vi "Test-SparkMax.vi"() -> ()   [LabVIEW 2023]
doc: "This VI implements the framework and scheduler for your robotics program. It should not be necessary to modify the framework. You are expected to add your code to the VIs called from Robot Main - the ones located in the Team Code folder within the project."
uses:
  Robot Global Data.vi
  <vilib>/Rock Robotics/WPI/DriverStation/WPI_DriverStationRobotMode2.ctl
  <vilib>/Rock Robotics/WPI/ThirdParty/REV Robotics/REVLib/Typedef/Spark MAX Limit Direction.ctl
  <vilib>/Rock Robotics/WPI/ThirdParty/REV Robotics/REVLib/Typedef/Spark MAX Limit Switch Polarity.ctl
panel:
  out "Loop Count":i32
  in  "Invert":bool
  in  "CAN Device Number":u8=1
  in  "Out-ut +/- 1.0":dbl
  out "Sensor Velocity  (REV/MIN)":dbl
  out "Sensor Position (REV)":dbl
  out "Hard Limit Rev":bool
  out "Hard Limit Fwd":bool
  in  "Rev Enabled":bool=TRUE
  in  "Rev Polarity":T1
  in  "Fwd Enabled":bool=TRUE
  in  "Fwd Polarity":T1
  in  "Finish":bool
  # "Set before starting\nProgram"
  # "Spark Max Test Program"
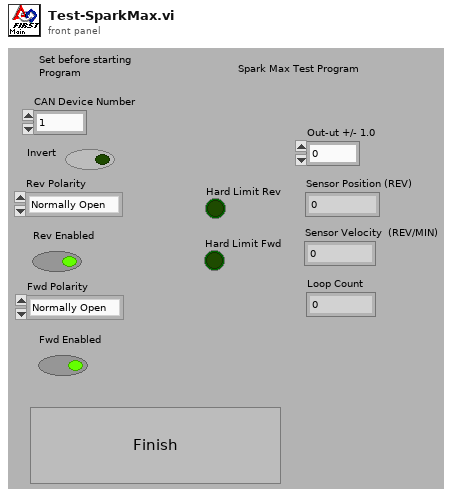
[diagram p1: front panel]
types:
  T1 = typedef "Spark MAX Limit Switch Polarity.ctl" = enum16{"Normally Open", "Normally Closed"}
  T2 = typedef "Spark MAX Limit Direction.ctl" = enum16{"Forward Limit", "Reverse Limit"}
  T3 = typedef "WPI_DriverStationRobotMode2.ctl" = enum16{"Autonomous Disabled", "Autonomous Enabled", "Teleop Disabled", "Teleop Enabled", "Disconnected", "Finish", "Test Disabled", "Test Enabled", "Emergency Stopped"}
  T4 = typedef "WPI_MotorControlDeviceRef.ctl" = cluster{"DeviceStatus":errorcluster, "Type":T5, "PWM":cluster{"PWM Channel":T6, "DeadBand":T7}, "CAN":cluster{"Device Number":u8, "SetOutput VI Ref":variant, "GetOutput VI Ref":variant, "Enable VI Ref":variant, "Disable VI Ref":variant, "Data":variant}, "Invert":bool, "DIO PWM":cluster{"PWM \"Enable\" Channel":T6, "DIOChannel":T8, "PWM Rate":dbl}}
  T5 = typedef "WPI_MotorControlType.ctl" = enum16{"PWM", "CAN", "DIO PWM"}
  T6 = typedef "FPGA_DIOPWMChannel.ctl" = enum8{"PWM 0", "PWM 1", "PWM 2", "PWM 3", "PWM 4", "PWM 5", "PWM 6", "PWM 7", "PWM 8", "PWM 9", "PWM MXP 0", "PWM MXP 1", "PWM MXP 2", "PWM MXP 3", "PWM MXP 4", "PWM MXP 5", "PWM MXP 6", "PWM MXP 7", "PWM MXP 8", "PWM MXP 9", "Invalid"}
  T7 = typedef "WPI_PWMDeadband.ctl" = cluster{"Name":string, "maxPositivePwm":i32, "minPositivePwm":i32, "centerPwm":i32, "maxNegativePwm":i32, "minNegativePwm":i32, "angularRange":u16}
  T8 = typedef "FPGA_DIOChannel.ctl" = enum8{"DIO 0", "DIO 1", "DIO 2", "DIO 3", "DIO 4", "DIO 5", "DIO 6", "DIO 7", "DIO 8", "DIO 9", "DIO MXP 0", "DIO MXP 1", "DIO MXP 2", "DIO MXP 3", "DIO MXP 4", "DIO MXP 5", "DIO MXP 6", "DIO MXP 7", "DIO MXP 8", "DIO MXP 9", "DIO MXP 10", "DIO MXP 11", "DIO MXP 12", "DIO MXP 13", "DIO MXP 14", "DIO MXP 15", "SPI Port CS1", "SPI Port CS2", "SPI Port CS3", "SPI Port MISO", "SPI Port MOSI", "Invalid"}
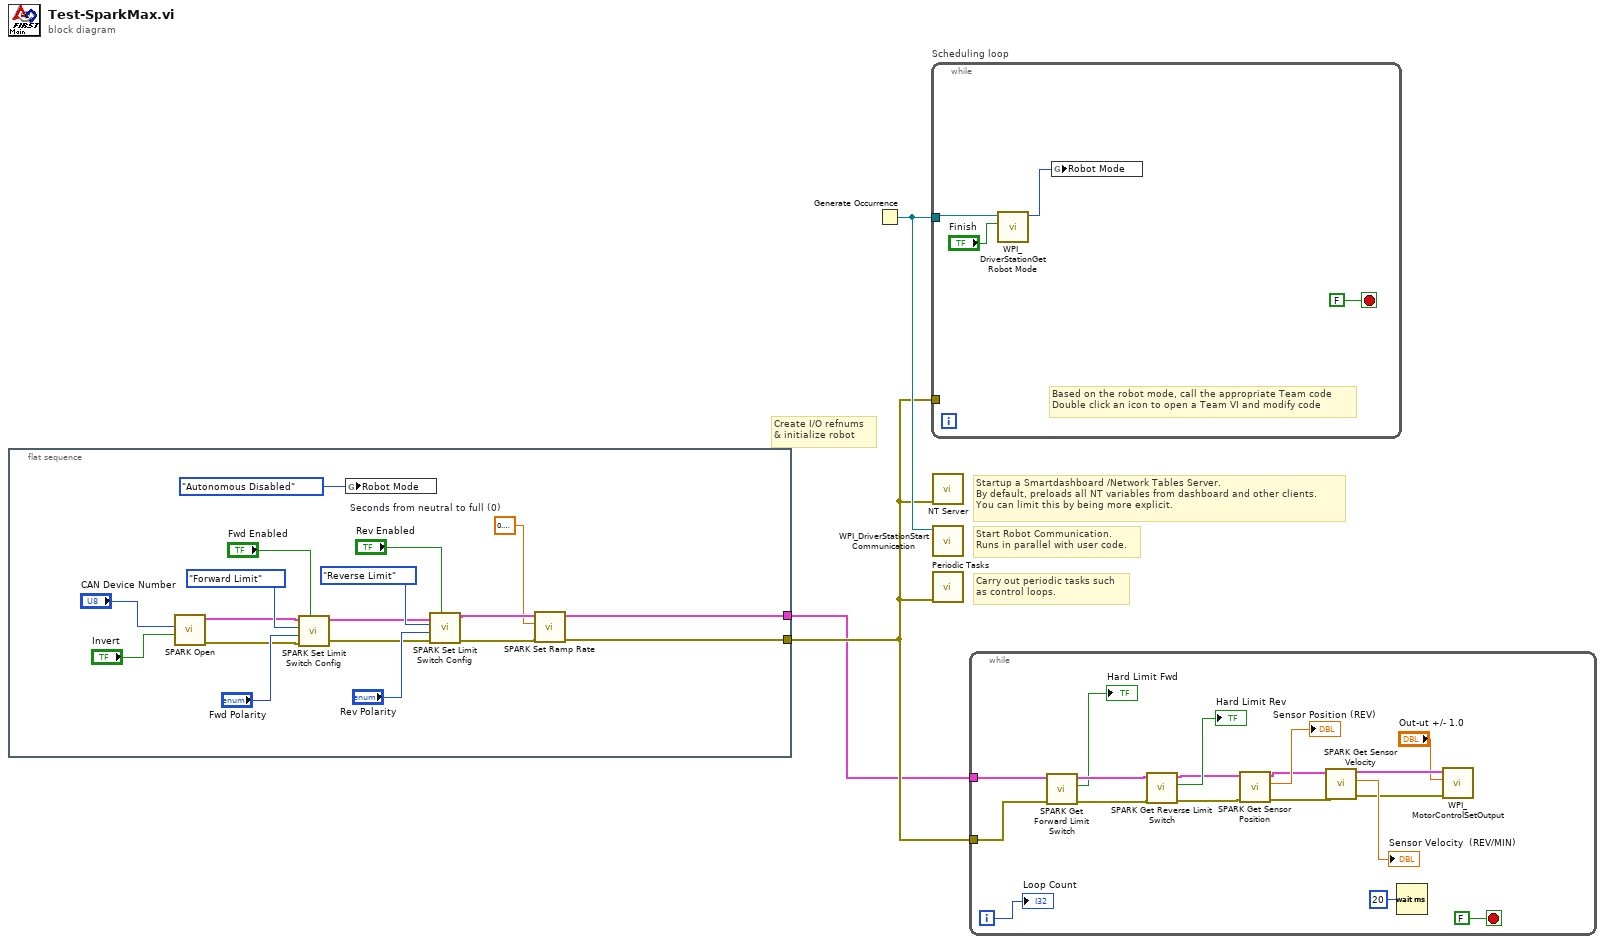
[diagram p0: block diagram]
diagram:
  # "Startup a Smartdashboard /Network Tables Server.\nBy default, preloads all NT variables from dashboard and other clients.\nYou can limit this by being more explicit."
  # "Carry out periodic tasks such\nas control loops."
  # "Create I/O refnums\n& initialize robot"
  # "Start Robot Communication.\nRuns in parallel with user code."
  n1 = flat-sequence {
    tunnel: [w7] -> w2
    tunnel: [w6] -> w1
    frame #0 {
      w9 = sgl 0.1  # Seconds from neutral to full (0)
      n2 = call <vilib>:"SPARK Open.vi"("Invert"="Invert", "Device Number"="CAN Device Number") -> ("error out"=w13:errorcluster, "MotorControlDeviceRef"=w14:T4)  [unwired: 8 in]
      n3 = call <vilib>:"SPARK Set Limit Switch Config.vi"("Enabled? (T)"="Fwd Enabled", "error in (no error)"=w13, "Polarity (Normally Open)"="Fwd Polarity", "Limit Switch"=Spark_MAX_Limit_Direction."Forward Limit", "MotorControlDeviceRef in"=w14) -> ("error out"=w11:errorcluster, "MotorControlDeviceRef out"=w12:T4)  [unwired: 5 in]
      n4 = global write "Robot Global Data.vi" "Robot Mode"(WPI_DriverStationRobotMode2."Autonomous Disabled" ("Robot Mode")) -> ()
      n5 = call <vilib>:"SPARK Set Limit Switch Config.vi"("Enabled? (T)"="Rev Enabled", "error in (no error)"=w11, "Polarity (Normally Open)"="Rev Polarity", "Limit Switch"=Spark_MAX_Limit_Direction."Reverse Limit", "MotorControlDeviceRef in"=w12) -> ("error out"=w8:errorcluster, "MotorControlDeviceRef out"=w10:T4)  [unwired: 5 in]
      n6 = call <vilib>:"SPARK Set Ramp Rate.vi"("error in (no error)"=w8, "Seconds from neutral to full (0)"=w9, "MotorControlDeviceRef in"=w10) -> ("error out"=w7:errorcluster, "MotorControlDeviceRef"=w6:T4)  [unwired: 7 in]
    }
  }
  n7 = Generate Occurrence() -> (w3:refnum<k4>)
  n8 = while "Scheduling loop" {
    tunnel: w3 -> [w25]
    tunnel: w2 -> [_]
    stop <- FALSE stop-if-true
    # "Based on the robot mode, call the appropriate Team code\nDouble click an icon to open a Team VI and modify code"
    n9 = call <vilib>:"WPI_DriverStationGet Robot Mode.vi"("Finish"="Finish", "DS Occurrence"=w25) -> ("Robot Mode"=w23:T3)  [unwired: 9 out]
    n10 = global write "Robot Global Data.vi" "Robot Mode"(w23) -> ()
  }
  n11 = call <vilib>:"NT Server.vi"("error in (no error)"=w2) -> ()  [unwired: 10 in, 1 out]
  n12 = call <vilib>:"WPI_DriverStationStart Communication.vi"("occurrence"=w3) -> ()  [unwired: 2 in, 9 out]
  n13 = call "Periodic Tasks.vi"("error in"=w2) -> ()  [unwired: 1 in, 10 out]
  n14 = while {
    tunnel: w2 -> [w40]
    tunnel: w1 -> [w41]
    i -> [w26]
    stop <- FALSE stop-if-true
    n15 = call <vilib>:"SPARK Get Forward Limit Switch.vi"("error in (no error)"=w40, "MotorControlDevRef in"=w41) -> ("error out"=w38:errorcluster, "Hard Limit Fwd"=→"Hard Limit Fwd":bool, "MotorControlDevRef out"=w39:T4)  [unwired: 6 in, 1 out]
    n16 = call <vilib>:"SPARK Get Reverse Limit Switch.vi"("error in (no error)"=w38, "MotorControlDevRef in"=w39) -> ("error out"=w35:errorcluster, "Hard Limit Rev"=→"Hard Limit Rev":bool, "MotorControlDevRef out"=w34:T4)  [unwired: 6 in, 1 out]
    n17 = call <vilib>:"SPARK Get Sensor Position.vi"("error in (no error)"=w35, "MotorControlDevRef in"=w34) -> ("error out"=w31:errorcluster, "Sensor Position"=→"Sensor Position (REV)":dbl, "MotorControlDevRef out"=w32:T4)  [unwired: 6 in, 1 out]
    n18 = call <vilib>:"SPARK Get Sensor Velocity.vi"("error in (no error)"=w31, "MotorControlDevRef in"=w32) -> ("error out"=w28:errorcluster, "Sensor Velocity"=→"Sensor Velocity  (REV/MIN)":dbl, "MotorControlDevRef out"=w30:T4)  [unwired: 6 in, 1 out]
    n19 = Wait (ms)(milliseconds to wait=u32 20) -> ()  [unwired: 1 out]
    n20 = call <vilib>:"WPI_MotorControlSetOutput.vi"("error in (no error)"=w28, "Output"="Out-ut +/- 1.0", "MotorControlDevRef"=w30) -> ()  [unwired: 6 in, 3 out]
    "Loop Count" <- w26
  }
